vi "非小号前百位数据整理.vi"() -> ()   [LabVIEW 2020]
uses:
  <vilib>/Utility/file.llb/Read Delimited Spreadsheet (string).vi
  <vilib>/Utility/file.llb/Write Delimited Spreadsheet (string).vi
panel:
  out "数组 3":string[][](array[string])
  out "数组 2":i32[](array[numeric])
  out "数组":string[](array[string])
  in  "file path (dialog if empty)":path caption="文件路径 （空时为对话框）"
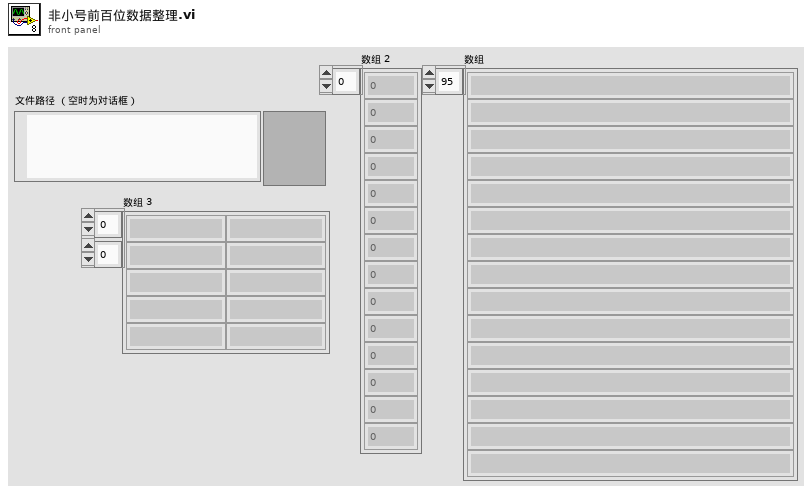
[diagram p1: front panel]
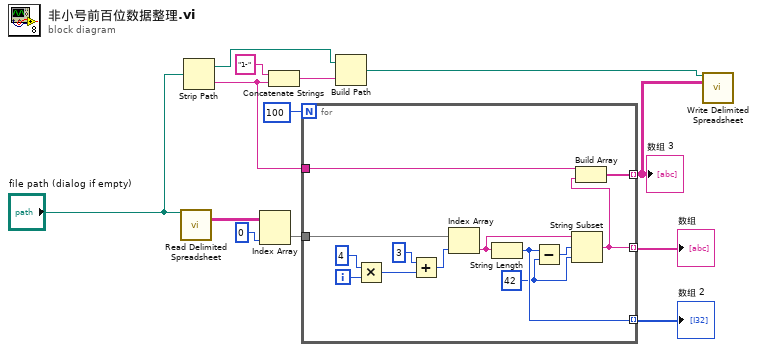
[diagram p0: block diagram]
diagram:
  n1 = call-poly <vilib>:"Read Delimited Spreadsheet.vi"("file path (dialog if empty)"="file path (dialog if empty)") -> ("all rows"=w12:string[][])  [unwired: 9 in, 5 out]
  n2 = Strip Path(path="file path (dialog if empty)") -> (stripped path=w4:path, name=w3:string)
  n3 = Index Array(array=w12, index (col)=0 ("禁用的索引 (列)")) -> (element=w10:string[])  [unwired: 1 in]
  n4 = Concatenate Strings("1-" ("字符串"), w3) -> (w5:string)
  n5 = for {
    N: 100 -> [_]
    tunnel: w10 -> [w26]
    tunnel: [w15] -> w9 mode=indexing
    tunnel: [w20] -> w8 mode=indexing
    tunnel: w3 -> [w16]
    tunnel: [w14] -> w2 mode=indexing
    i -> [w25]
    w18 = 42 ("y")
    n6 = Multiply(x=4, y=w25) -> (x*y=w23:i32)
    n7 = Add(x=3, y=w23) -> (x+y=w21:i32)
    n8 = Index Array(array=w26, index=w21) -> (element=w19:string)
    n9 = String Length(string=w19) -> (length=w20:i32)
    n10 = Subtract(x=w20, y=w18) -> (x-y=w17:i32)
    n11 = String Subset(string=w19, offset (0)=w17, length (rest)=w18) -> (substring=w15:string)
    n12 = Build Array(w16, w15) -> (w14:string[])
  }
  "数组" <- w9
  "数组 2" <- w8
  "数组 3" <- w2
  n13 = Build Path(base path=w4, name or relative path=w5) -> (appended path=w1:path)
  n14 = call-poly <vilib>:"Write Delimited Spreadsheet.vi"("file path (dialog if empty)"=w1, "2D data"=w2) -> ()  [unwired: 12 in, 2 out]
